vi "pop upper panel.vi"(1 "error in (no error)":errorcluster, 2 "Tool Selection":T1, 3 "pop vi":bool, 4 "Sub Panel":refnum<vi>) -> (0 "error out":errorcluster)   [LabVIEW 2016, in "main.lvlib"]
doc: "pop upper panel.vi \"pops\" out Tools VI that is currently in \nupper sub-panel making it a stand-alone VI."
uses:
  main.lvlib
  tool selection.ctl
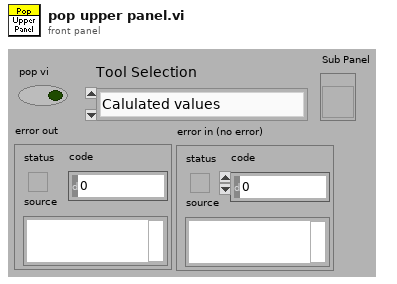
[diagram p1: front panel]
types:
  T1 = typedef "main.lvlib/tool selection.ctl" = enum16{"Calulated values", "Scale", "Currents", "Injector magnet", "Terminal Voltage", "Source BPM", "Vacuum", "Flat Top", "Zero Values", "Terminal Control", "Scan Injector"}
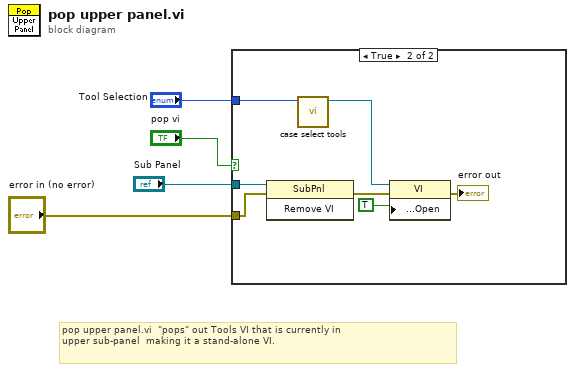
[diagram p0: block diagram]
diagram:
  # "pop upper panel.vi  \"pops\" out Tools VI that is currently in \nupper sub-panel  making it a stand-alone VI."
  n1 = case shown="True" "pop vi" {
    tunnel: "Sub Panel" -> [_ w11]
    tunnel: "Tool Selection" -> [_ w5]
    tunnel: "error in (no error)" -> [_ w8]
    frame False {
    }
    frame True {
      n2 = invoke class="SubPnl" method="Remove VI"(reference=w11, error in=w8) -> (error out=w10:errorcluster)  [unwired: 1 in, 2 out]
      n3 = call "case select tools.vi"("Tool Selection"=w5) -> ("VI out"=w6:refnum<vi>)  [unwired: 10 in]
      n4 = property class="VI"(reference=w6, error in=w10, "Front Panel.Open"=TRUE ("Front Panel Window:Open")) -> (error out=→"error out":errorcluster)  [unwired: 1 out]
    }
  }
